vi "calibratedSafeStates.vi"(8 "error in (no error)":errorcluster, 11 "RfOutputChannel in":refnum<class "RfOutputChannel.lvclass">) -> (0 "error out":errorcluster, 2 "OutputDefaults":T1, 3 "RfOutputChannel out":refnum<class "RfOutputChannel.lvclass">)   [LabVIEW 2009, in "Tools.lvlib" / "DatabaseHelpers.lvlib" / "RfOutputChannel.lvclass"]
uses:
  RfOutputChannel.lvclass
  RfOutputChannel.lvclass/RfOutputChannel.ctl
  Channel.lvclass
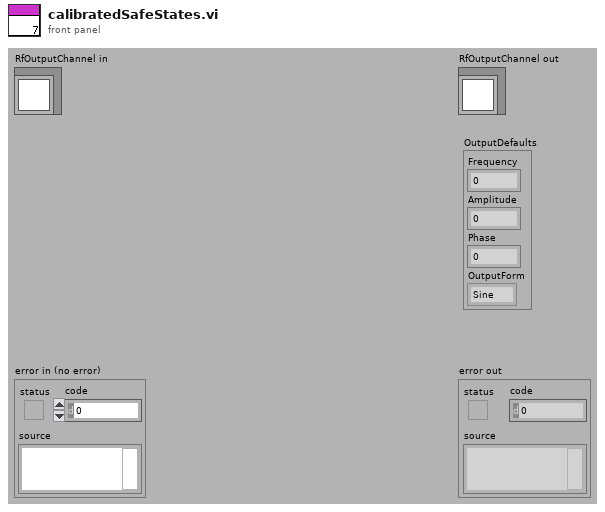
[diagram p1: front panel]
types:
  T1 = cluster{"Frequency":dbl, "Amplitude":dbl, "Phase":dbl, "OutputForm":enum16{"Sine", "Square", "Triangle", "Arbitrary"}}
  T2 = enum16{"Sine", "Square", "Triangle", "Arbitrary"}
  T3 = cluster{"state_name":string, "value":cluster{"frequency":string, "amplitude":string, "phase":string}}[]
  T4 = cluster{"frequency":string, "amplitude":string, "phase":string}
  T5 = cluster{"freq":dbl, "Amplitude":dbl, "Phase":dbl, "OutputForm":enum16{"Sine", "Square", "Triangle", "Arbitrary"}}
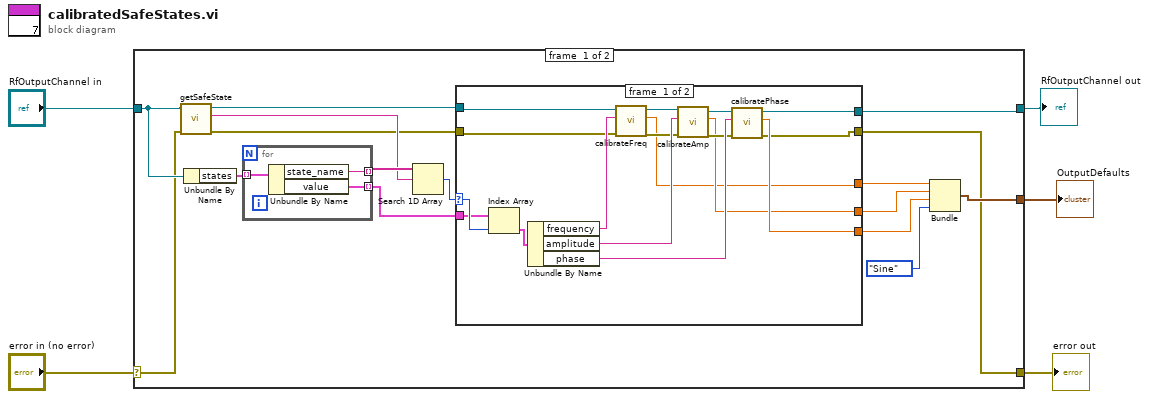
[diagram p0: block diagram]
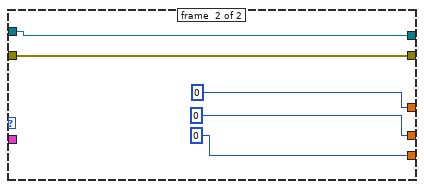
[diagram p2: hidden frame]
diagram:
  n1 = case shown="No Error" "error in (no error)" {
    selector: "error in (no error)" -> [w19 w48]
    tunnel: [w6 w48] -> w4
    tunnel: [w12 w47] -> w2
    tunnel: "RfOutputChannel in" -> [w20 w47]
    tunnel: [w8 _] -> w1
    frame #0 {
      n2 = call "getSafeState.vi"("error in (no error)"=w19, "Channel.lvclass in"=w20) -> ("error out"=w14:errorcluster, "safe_state"=w17:string, "Channel.lvclass out"=w15:refnum<class "RfOutputChannel.lvclass">)  [unwired: 7 in]
      n3 = Unbundle By Name(w20) -> ("states"=w21:T3)
      n4 = for {
        tunnel: w21 -> [w46] mode=indexing
        tunnel: [w45] -> w18 mode=indexing
        tunnel: [w44] -> w13 mode=indexing
        n5 = Unbundle By Name(w46) -> ("state_name"=w45:string, "value"=w44:T4)
      }
      n6 = Search 1D Array(1D array=w18, element=w17) -> (index of element=w16:i32)  [unwired: 1 in]
      n7 = case shown="0, Default" w16 {
        selector: w16 -> [w38 _]
        tunnel: w15 -> [w35 w40]
        tunnel: w14 -> [w33 w39]
        tunnel: w13 -> [w37 _]
        tunnel: [w26 w40] -> w12
        tunnel: [w25 0] -> w9
        tunnel: [w24 0] -> w10
        tunnel: [w23 0] -> w11
        tunnel: [w22 w39] -> w6
        frame #0 {
          n8 = Index Array(array=w37, index=w38) -> (element=w36:T4)
          n9 = Unbundle By Name(w36) -> ("frequency"=w34:string, "amplitude"=w31:string, "phase"=w28:string)
          n10 = call "calibrateFreq.vi"("error in (no error)"=w33, "value"=w34, "RfOutputChannel in"=w35) -> ("error out"=w30:errorcluster, "freq"=w23:dbl, "RfOutputChannel out"=w32:refnum<class "RfOutputChannel.lvclass">)  [unwired: 6 in]
          n11 = call "calibrateAmp.vi"("error in (no error)"=w30, "value"=w31, "RfOutputChannel in"=w32) -> ("error out"=w27:errorcluster, "Amplitude"=w24:dbl, "RfOutputChannel out"=w29:refnum<class "RfOutputChannel.lvclass">)  [unwired: 6 in]
          n12 = call "calibratePhase.vi"("error in (no error)"=w27, "value"=w28, "RfOutputChannel in"=w29) -> ("error out"=w22:errorcluster, "Phase"=w25:dbl, "RfOutputChannel out"=w26:refnum<class "RfOutputChannel.lvclass">)  [unwired: 6 in]
        }
        frame #1 {
        }
      }
      n13 = Bundle("freq"=w11, "Amplitude"=w10, "Phase"=w9, "OutputForm"=T2."Sine") -> (w8:T5)  [unwired: 1 in]
    }
    frame #1 {
    }
  }
  "error out" <- w4
  "RfOutputChannel out" <- w2
  "OutputDefaults" <- w1
